vi "main.vi"() -> ()   [LabVIEW 2024]
uses:
  <vilib>/National Instruments/NI Super Simple Neural Networks/Neural Network.lvclass
panel:
  out "image 28x28":u8[][](graph)
  out "new picture":picture
  out "Rezultat":string
  in  "pen 2":T1={"Width"=10, "Style"=enum."Solid"}
  in  "stop":bool
  in  "Refresh Button":bool
  out "Clasificare clase":cluster{string, "Numeric Control":dbl}[](array[cluster])
  out "picture":picture
  out "pen":T1={"Width"=1, "Style"=enum."Solid"}
  in  "NN-Configuratie":path
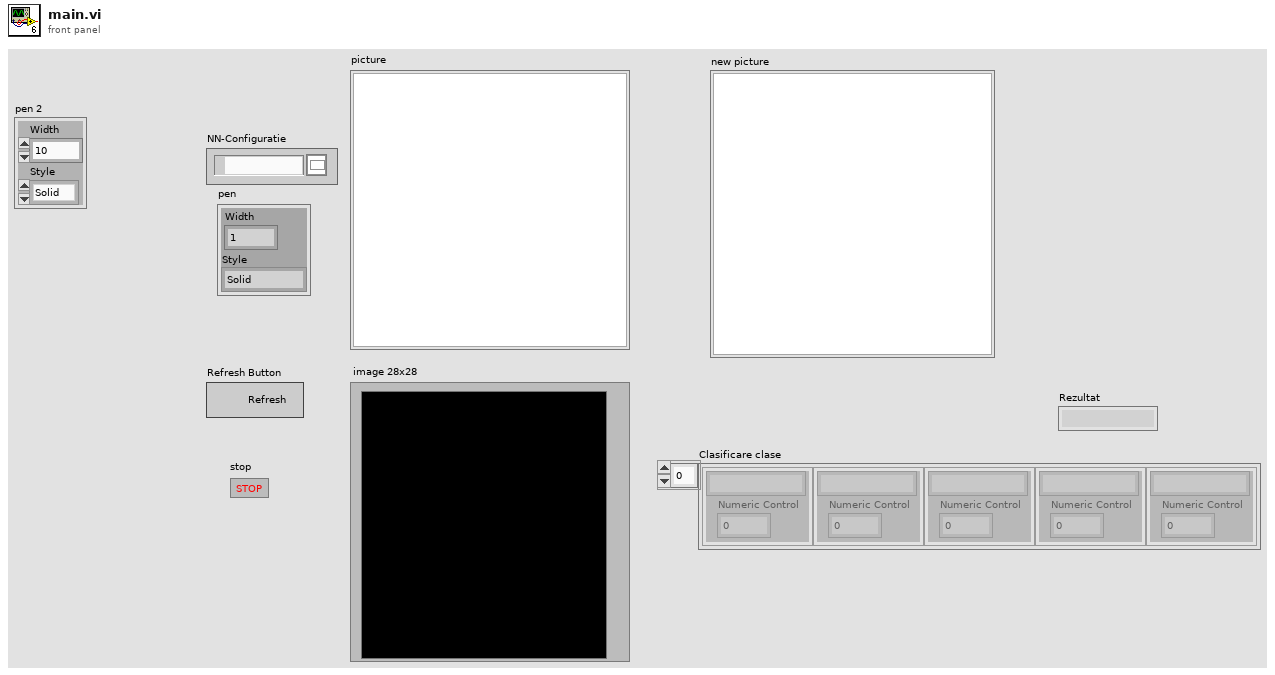
[diagram p1: front panel]
types:
  T1 = cluster{"Width":u16, "Style":enum32{"Solid", "Dash", "Dot", "DashDot", "DashDotDot"}}
  T2 = enum16{"Normalizare [0,1]", "Normalizare[-1,1]", "Fara normalizare"}
  T3 = cluster{"left":i16, "top":i16, "right":i16, "bottom":i16}
  T4 = typedef "LVMouseTypeDef.ctl" = cluster{"Mouse Position":cluster{"X":i32, "Y":i32}, "Mouse Modifiers":cluster{"Button Down":bool, "Shift Mod":bool, "Menu Mod":bool, "Option Mod":bool}}
  T5 = typedef "imagedata.ctl" = cluster{"image type":i32, "image depth":i32, "image":u8[], "mask":u8[], "colors":u32[], "Rectangle":cluster{"left":i16, "top":i16, "right":i16, "bottom":i16}}
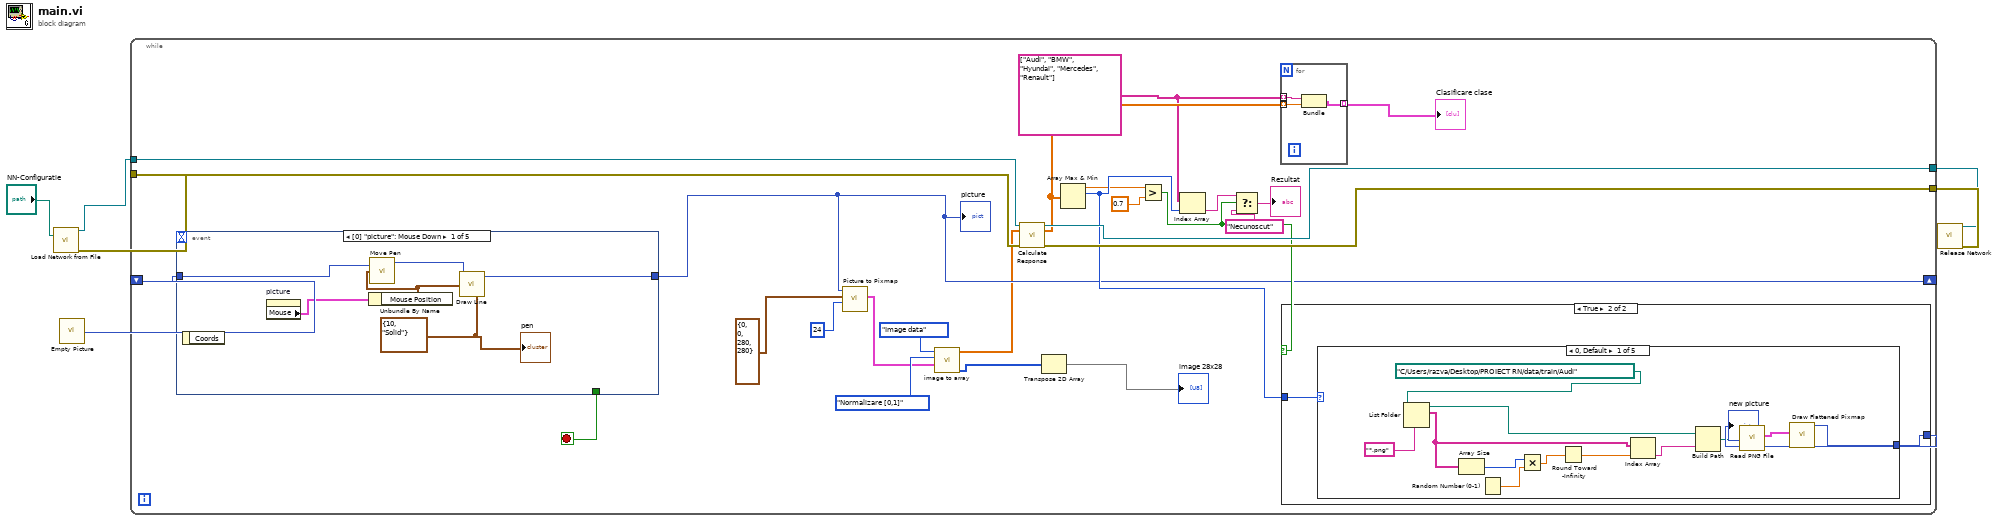
[diagram p0: block diagram]
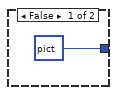
[diagram p2: hidden frame]
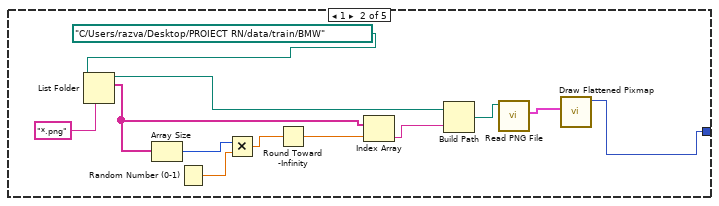
[diagram p3: hidden frame]
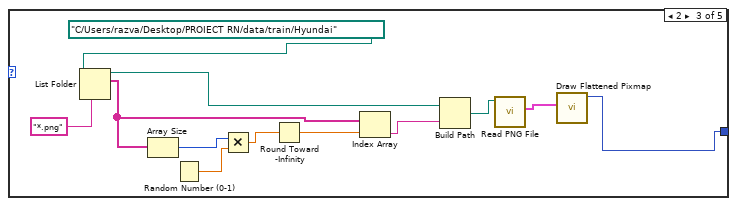
[diagram p4: hidden frame]
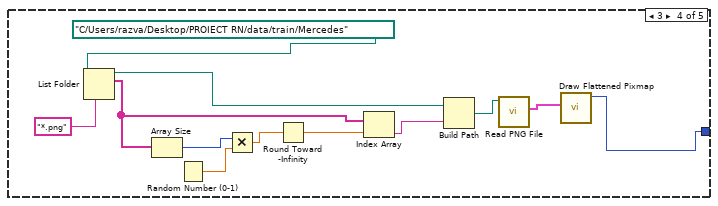
[diagram p5: hidden frame]
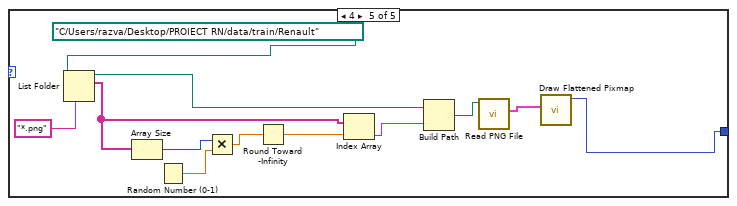
[diagram p6: hidden frame]
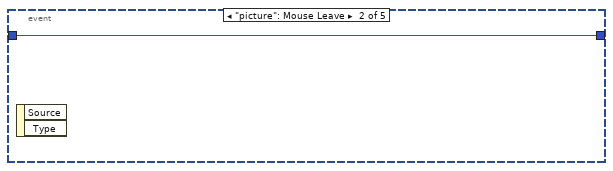
[diagram p7: hidden frame]
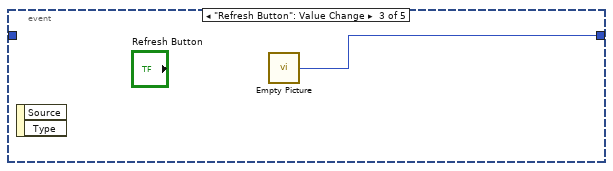
[diagram p8: hidden frame]
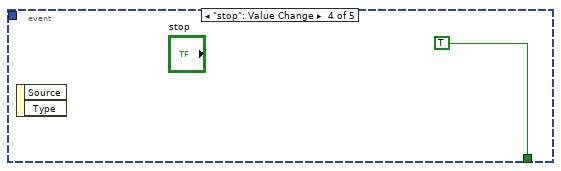
[diagram p9: hidden frame]
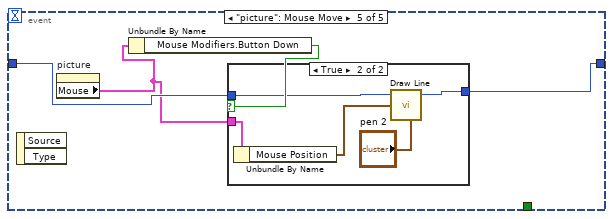
[diagram p10: hidden frame]
diagram:
  n1 = call <vilib>:"Load Network from File.vi"("File Path (dialog)"="NN-Configuratie") -> ("Neural Network Out"=w3:refnum<class "Neural Network.lvclass">, "Error Out"=w4:errorcluster)  [unwired: 11 in, 2 out]
  n2 = call "Empty Picture"() -> ("empty picture"=w5:picture)
  n3 = while {
    shift-right: [w15] -> _
    shift-left: w5 -> [w32]
    tunnel: w4 -> [w31]
    tunnel: w3 -> [w30]
    tunnel: [w27] -> w2
    tunnel: [w26] -> w1
    stop <- w29 stop-if-true
    w20 = string[] ["Audi", "BMW", "Hyundai", "Mercedes", "Renault"]
    n4 = event shown="[0] \"picture\": Mouse Down" {
      selector: _ -> [_ _ _ _ _]
      dyn-events: _ -> [_ _ _ _ _]
      timeout: _ -> [_ _ _ _ _]
      tunnel: w32 -> [w104 w105 _ _ w110]
      tunnel: [w102 w105 w106 _ w109] -> w15
      tunnel: [_ _ _ TRUE _] -> w29
      event "picture": Mouse Down {
        w101 = T1 {"Width"=10, "Style"=enum."Solid"} ("pen")
        n5 = event-data() -> ()  [unwired: 1 in, 1 out]
        n6 = property on="picture" class="Pict"() -> ("Mouse"=w100:T4)  [unwired: 2 in, 2 out]
        n7 = Unbundle By Name(w100) -> ("Mouse Position"=w99:cluster{"X":i32, "Y":i32})
        n8 = call <vilib>:"Move Pen.vi"("new position"=w99, "picture"=w104) -> ("new picture"=w103:picture)  [unwired: 3 in]
        n9 = call <vilib>:"Draw Line.vi"("picture"=w103, "end point"=w99, "pen"=w101) -> ("new picture"=w102:picture)  [unwired: 6 in]
        "pen" <- w101
      }
      event "picture": Mouse Leave {
        n10 = event-data() -> ()  [unwired: 1 in, 2 out]
      }
      event "Refresh Button": Value Change {
        n11 = event-data() -> ()  [unwired: 1 in, 2 out]
        n12 = call "Empty Picture"() -> ("empty picture"=w106:picture)
      }
      event "stop": Value Change {
        n13 = event-data() -> ()  [unwired: 1 in, 2 out]
      }
      event "picture": Mouse Move {
        n14 = event-data() -> ()  [unwired: 1 in, 2 out]
        n15 = property on="picture" class="Pict"() -> ("Mouse"=w108:T4)  [unwired: 2 in, 2 out]
        n16 = Unbundle By Name(w108) -> ("Mouse Modifiers.Button Down"=w111:bool)
        n17 = case shown="True" w111 {
          tunnel: w110 -> [w112 w115]
          tunnel: w108 -> [_ w113]
          tunnel: [w112 w114] -> w109
          frame False {
          }
          frame True {
            n18 = Unbundle By Name(w113) -> ("Mouse Position"=w116:cluster{"X":i32, "Y":i32})
            n19 = call <vilib>:"Draw Line.vi"("picture"=w115, "end point"=w116, "pen"="pen 2") -> ("new picture"=w114:picture)  [unwired: 6 in]
          }
        }
      }
    }
    "picture" <- w15
    n20 = call <vilib>:"Picture to Pixmap.vi"("depth"=24, "rect"=T3 {"left"=0, "top"=0, "right"=280, "bottom"=280}, "picture"=w15) -> ("image data"=w9:T5)  [unwired: 7 in, 1 out]
    n21 = call "image to array.vi"("image data"=w9, "Normalizare"=T2."Normalizare [0,1]", "Image type"=enum16{"Image file (png)", "Image data"}."Image data") -> ("Image 28x28"=w8:u8[][], "Image 1d Array"=w7:dbl[])  [unwired: 4 in, 3 out]
    n22 = call <vilib>:"Calculate Response.vi"("Neural Network In"=w30, "Inputs"=w7, "Error In"=w31) -> ("Neural Network Out"=w26:refnum<class "Neural Network.lvclass">, "Outputs"=w25:dbl[], "Error Out"=w27:errorcluster)  [unwired: 10 in]
    n23 = Transpose 2D Array(2D array=w8) -> (transposed array=→"image 28x28":u8[][])
    n24 = Array Max & Min(array=w25) -> (max value=w16:dbl, max index (indices)=w17:i32)  [unwired: 2 out]
    n25 = Greater?(x=w16, y=0.7) -> (0:w18:bool)
    n26 = Index Array(array=w20, index=w17) -> (element=w23:string)
    n27 = Select(t=w23, s=w18, f="Necunoscut") -> (s? t:f=→"Rezultat":string)
    n28 = for {
      tunnel: w25 -> [w98] mode=indexing
      tunnel: w20 -> [w97] mode=indexing
      tunnel: [w96] -> w28 mode=indexing
      n29 = Bundle(w97, "Numeric Control"=w98) -> (w96:cluster{string, "Numeric Control":dbl})  [unwired: 1 in]
    }
    "Clasificare clase" <- w28
    n30 = case shown="True" w18 {
      tunnel: [picture data[5B] ("new picture") w35] -> w19
      tunnel: w17 -> [_ w34]
      frame False {
      }
      frame True {
        n31 = case shown="0, Default" w34 {
          tunnel: [w37 w49 w61 w73 w85] -> w35
          frame 0, Default {
            n32 = List Folder(path=path "C:/Users/razva/Desktop/PROIECT RN/data/train/Audi", pattern="*.png") -> (path out=w41:path, filenames=w36:string[])  [unwired: 2 in, 2 out]
            n33 = Array Size(array=w36) -> (size(s)=w45:i32)
            n34 = Random Number (0-1)() -> (number: 0 to 1=w44:dbl)
            n35 = Multiply(x=w45, y=w44) -> (x*y=w43:dbl)
            n36 = Round Toward -Infinity(1:w43) -> (0:w42:dbl)
            n37 = Index Array(array=w36, index=w42) -> (element=w40:string)
            n38 = Build Path(base path=w41, name or relative path=w40) -> (appended path=w39:path)
            n39 = call <vilib>:"Read PNG File.vi"("path to PNG file"=w39) -> ("image data"=w38:T5)  [unwired: 8 in, 2 out]
            n40 = call <vilib>:"Draw Flattened Pixmap.vi"("image data"=w38) -> ("new picture"=w37:picture)  [unwired: 8 in]
          }
          frame 1 {
            n41 = List Folder(path=path "C:/Users/razva/Desktop/PROIECT RN/data/train/BMW", pattern="*.png") -> (path out=w53:path, filenames=w48:string[])  [unwired: 2 in, 2 out]
            n42 = Array Size(array=w48) -> (size(s)=w57:i32)
            n43 = Random Number (0-1)() -> (number: 0 to 1=w56:dbl)
            n44 = Multiply(x=w57, y=w56) -> (x*y=w55:dbl)
            n45 = Round Toward -Infinity(1:w55) -> (0:w54:dbl)
            n46 = Index Array(array=w48, index=w54) -> (element=w52:string)
            n47 = Build Path(base path=w53, name or relative path=w52) -> (appended path=w51:path)
            n48 = call <vilib>:"Read PNG File.vi"("path to PNG file"=w51) -> ("image data"=w50:T5)  [unwired: 8 in, 2 out]
            n49 = call <vilib>:"Draw Flattened Pixmap.vi"("image data"=w50) -> ("new picture"=w49:picture)  [unwired: 8 in]
          }
          frame 2 {
            n50 = List Folder(path=path "C:/Users/razva/Desktop/PROIECT RN/data/train/Hyundai", pattern="*.png") -> (path out=w65:path, filenames=w60:string[])  [unwired: 2 in, 2 out]
            n51 = Array Size(array=w60) -> (size(s)=w69:i32)
            n52 = Random Number (0-1)() -> (number: 0 to 1=w68:dbl)
            n53 = Multiply(x=w69, y=w68) -> (x*y=w67:dbl)
            n54 = Round Toward -Infinity(1:w67) -> (0:w66:dbl)
            n55 = Index Array(array=w60, index=w66) -> (element=w64:string)
            n56 = Build Path(base path=w65, name or relative path=w64) -> (appended path=w63:path)
            n57 = call <vilib>:"Read PNG File.vi"("path to PNG file"=w63) -> ("image data"=w62:T5)  [unwired: 8 in, 2 out]
            n58 = call <vilib>:"Draw Flattened Pixmap.vi"("image data"=w62) -> ("new picture"=w61:picture)  [unwired: 8 in]
          }
          frame 3 {
            n59 = List Folder(path=path "C:/Users/razva/Desktop/PROIECT RN/data/train/Mercedes", pattern="*.png") -> (path out=w77:path, filenames=w72:string[])  [unwired: 2 in, 2 out]
            n60 = Array Size(array=w72) -> (size(s)=w81:i32)
            n61 = Random Number (0-1)() -> (number: 0 to 1=w80:dbl)
            n62 = Multiply(x=w81, y=w80) -> (x*y=w79:dbl)
            n63 = Round Toward -Infinity(1:w79) -> (0:w78:dbl)
            n64 = Index Array(array=w72, index=w78) -> (element=w76:string)
            n65 = Build Path(base path=w77, name or relative path=w76) -> (appended path=w75:path)
            n66 = call <vilib>:"Read PNG File.vi"("path to PNG file"=w75) -> ("image data"=w74:T5)  [unwired: 8 in, 2 out]
            n67 = call <vilib>:"Draw Flattened Pixmap.vi"("image data"=w74) -> ("new picture"=w73:picture)  [unwired: 8 in]
          }
          frame 4 {
            n68 = List Folder(path=path "C:/Users/razva/Desktop/PROIECT RN/data/train/Renault", pattern="*.png") -> (path out=w89:path, filenames=w84:string[])  [unwired: 2 in, 2 out]
            n69 = Array Size(array=w84) -> (size(s)=w93:i32)
            n70 = Random Number (0-1)() -> (number: 0 to 1=w92:dbl)
            n71 = Multiply(x=w93, y=w92) -> (x*y=w91:dbl)
            n72 = Round Toward -Infinity(1:w91) -> (0:w90:dbl)
            n73 = Index Array(array=w84, index=w90) -> (element=w88:string)
            n74 = Build Path(base path=w89, name or relative path=w88) -> (appended path=w87:path)
            n75 = call <vilib>:"Read PNG File.vi"("path to PNG file"=w87) -> ("image data"=w86:T5)  [unwired: 8 in, 2 out]
            n76 = call <vilib>:"Draw Flattened Pixmap.vi"("image data"=w86) -> ("new picture"=w85:picture)  [unwired: 8 in]
          }
        }
      }
    }
    "new picture" <- w19
  }
  n77 = call <vilib>:"Release Network.vi"("Neural Network"=w1, "Error In"=w2) -> ()  [unwired: 13 in, 1 out]
